vi "LoggerGlobal.vi"() -> ()   [LabVIEW 2020, in "Logger.lvlib"]
uses:
  Logger.lvlib
  Event.ctl
panel:
  in  "Path":path
  out "Logger Queue":refnum<queue>
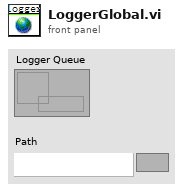
[diagram p1: front panel]
diagram:
